vi "Execute.Initialize.vi"(8 "error in (no error)":errorcluster, 11 "Cluster":T1) -> (0 "error out":errorcluster)   [LabVIEW 2013, in "Simple Sequence Editor.lvlib"]
uses:
  Simple Sequence Editor.lvlib
  Types/Execuction.StateVariables.ctl
  <vilib>/NI Veristand/Execution/SequenceExecutionInterface/Stimulus Profile Session Ref.ctl
  NationalInstruments.VeriStand.ClientAPI
  <vilib>/NI Veristand/Execution/Workspace/SystemStateRegEventRef.ctl
  <vilib>/NI Veristand/Execution/Workspace/SystemStateEventRef.ctl
  <vilib>/NI Veristand/Execution/Workspace/WorkspaceAPI.ctl
  Types/Execute.PreviewMode.ctl
  Constants.vi
  <vilib>/NI Veristand/Execution/Workspace/NI_VS Workspace ExecutionAPI.lvlib
  <vilib>/NI Veristand/Execution/SequenceExecutionInterface/NI_VS Sequence Execution Interface.lvlib
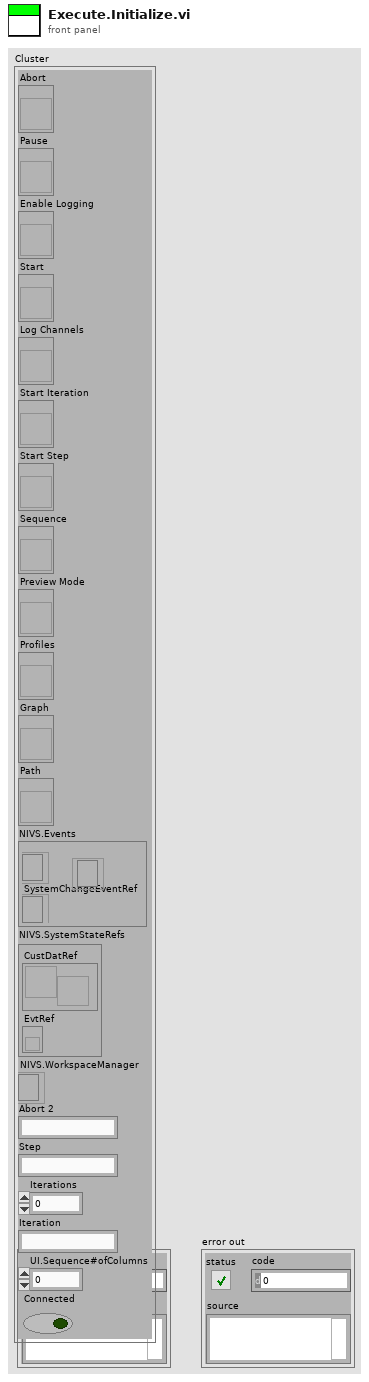
[diagram p1: front panel]
types:
  T1 = typedef "Simple Sequence Editor.lvlib/Execuction.StateVariables.ctl" = cluster{"Abort":refnum<vi>, "Pause":refnum<vi>, "Enable Logging":refnum<vi>, "Start":refnum<vi>, "Log Channels":refnum<vi>, "Start Iteration":refnum<vi>, "Start Step":refnum<vi>, "Sequence":refnum<vi>, "Preview Mode":refnum<vi>, "Profiles":refnum<vi>, "Graph":refnum<vi>, "Path":refnum<vi>, "NIVS.Events":cluster{"Complete":refnum<event-registration>, "NIVS.Workspace Event":refnum<event-registration>, "SystemChangeEventRef":T2}, "NIVS.SystemStateRefs":T3, "NIVS.WorkspaceManager":T4, "Abort 2":string, "Step":string, "Iterations":u32, "Iteration":string, "UI.Sequence#ofColumns":i32, "Connected":bool}
  T2 = typedef "NI_VS Workspace ExecutionAPI.lvlib/SystemStateRegEventRef.ctl" = refnum<event-registration>
  T3 = typedef "NI_VS Workspace ExecutionAPI.lvlib/SystemStateEventRef.ctl" = cluster{"CustDatRef":refnum<user-event>, "EvtRef":refnum<k27>}
  T4 = typedef "NI_VS Workspace ExecutionAPI.lvlib/WorkspaceAPI.ctl" = refnum<k24>
  T5 = enum8{"Enabled", "Disabled", "Disabled and Grayed Out"}
  T6 = typedef "Simple Sequence Editor.lvlib/Execute.PreviewMode.ctl" = enum8{"Graph", "Table"}
  T7 = enum16{"Channels (No System Channel)", "Aliases", "All"}
  T8 = typedef "LVBoundsTypeDef.ctl" = cluster{"Width":u32, "Height":u32}
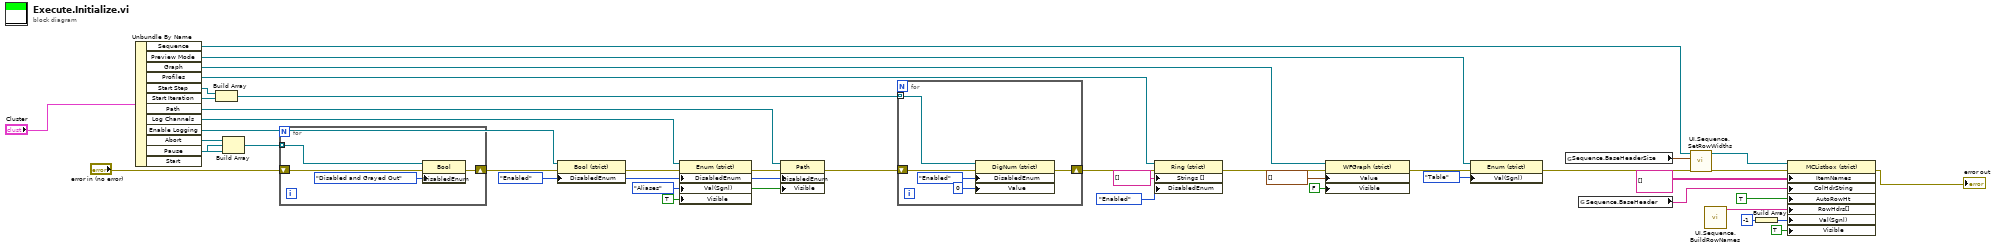
[diagram p0: block diagram]
diagram:
  w1 = TRUE ("Visible")
  w4 = T5."Enabled" ("Disabled")
  n1 = Unbundle By Name("Cluster") -> ("Sequence"=w43:refnum<vi>, "Preview Mode"=w29:refnum<vi>, "Graph"=w26:refnum<vi>, "Profiles"=w23:refnum<vi>, "Start Step"=w20:refnum<vi>, "Start Iteration"=w19:refnum<vi>, "Path"=w5:refnum<vi>, "Log Channels"=w16:refnum<vi>, "Enable Logging"=w15:refnum<vi>, "Abort"=w10:refnum<vi>, "Pause"=w11:refnum<vi>, "Start"=w12:refnum<vi>)
  n2 = Build Array(w20, w19) -> (w21:refnum<vi>[])
  n3 = Build Array(w10, w11, w12) -> (w13:refnum<vi>[])
  n4 = for {
    tunnel: w13 -> [w47] mode=indexing
    shift-right: [w45] -> w14
    shift-left: "error in (no error)" -> [w44]
    n5 = property class="Bool"(reference=w47, error in=w44, "DisabledEnum"=T5."Disabled and Grayed Out" ("Disabled")) -> (error out=w45:errorcluster)  [unwired: 1 out]
  }
  n6 = property class="Bool (strict)"(reference=w15, error in=w14, "DisabledEnum"=w4) -> (error out=w17:errorcluster)  [unwired: 1 out]
  n7 = property class="Enum (strict)"(reference=w16, error in=w17, "DisabledEnum"=w4, "Val(Sgnl)"=T7."Aliases" ("Value (Signaling)"), "Visible"=w1) -> (error out=w3:errorcluster)  [unwired: 1 out]
  n8 = property class="Path"(reference=w5, error in=w3, "DisabledEnum"=w4, "Visible"=w1) -> (error out=w2:errorcluster)  [unwired: 1 out]
  n9 = for {
    tunnel: w21 -> [w52] mode=indexing
    shift-right: [w50] -> w22
    shift-left: w2 -> [w49]
    n10 = property class="DigNum (strict)"(reference=w52, error in=w49, "DisabledEnum"=T5."Enabled" ("Disabled"), "Value"=u32 0) -> (error out=w50:errorcluster)  [unwired: 1 out]
  }
  n11 = property class="Ring (strict)"(reference=w23, error in=w22, "Strings []"=string[] [], "DisabledEnum"=T5."Enabled" ("Disabled")) -> (error out=w25:errorcluster)  [unwired: 1 out]
  n12 = property class="WFGraph (strict)"(reference=w26, error in=w25, "Value"=waveform(dbl)[] [], "Visible"=FALSE) -> (error out=w30:errorcluster)  [unwired: 1 out]
  n13 = property class="Enum (strict)"(reference=w29, error in=w30, "Val(Sgnl)"=Execute.PreviewMode."Table" ("View")) -> (error out=w41:errorcluster)  [unwired: 1 out]
  n14 = global read "Constants.vi" "Sequence.BaseHeaderSize"() -> (w36:T8[])
  n15 = global read "Constants.vi" "Sequence.BaseHeader"() -> (w35:string[])
  n16 = call "UI.Sequence.SetRowWidths.vi"("error in (no error)"=w41, "CellSize"=w36, "UI.SequenceRef"=w43) -> ("error out"=w40:errorcluster, "UI.SequenceRef"=w33:refnum<vi>)  [unwired: 7 in]
  n17 = call "UI.Sequence.BuildRowNames.vi"() -> ("Row Headings"=w38:string[])  [unwired: 11 in]
  n18 = Build Array(-1 ("Value")) -> (w37:i32[])
  n19 = property class="MCListbox (strict)"(reference=w33, error in=w40, "ItemNames"=string[][] [] ("Item Names"), "ColHdrString"=w35, "AutoRowHt"=TRUE ("Autosizing Row Height"), "RowHdrs[]"=w38, "Val(Sgnl)"=w37, "Visible"=TRUE) -> (error out=→"error out":errorcluster)  [unwired: 1 out]
